vi "Publish.vi"(7 "Event Name":string, 8 "error in (no error)":errorcluster, 9 "Main Message":string="This text isn't used for sms", 10 "Subject":string="This is a test of the blah blah blah message system", 11 "connection in":T1) -> (0 "error out":errorcluster, 3 "connection out":T1)   [LabVIEW 2014, in "FRCts20_SNS.lvlib"]
uses:
  FRCts20_SNS.lvlib
  <vilib>/National Instruments/NI Amazon Web Services (AWS) Toolkit for LabVIEW/SNS/VI Source/AWS SNS Class/AWS_SNS.lvclass
  <vilib>/National Instruments/NI Amazon Web Services (AWS) Toolkit for LabVIEW/S3/vi source/Typedefs/AMZ_S3_AWS Credentials.ctl
  <vilib>/National Instruments/NI Amazon Web Services (AWS) Toolkit for LabVIEW/S3/vi source/LV Interface for Amazon S3.lvlib
  <vilib>/addons/database/NI_Database_API.lvlib
  <vilib>/addons/database/Connection.llb/DB Tools Open Connec (String).vi
  <vilib>/addons/database/Connection.llb/Conn ObjectReference.ctl
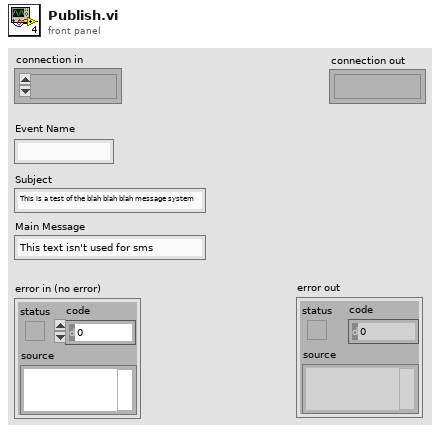
[diagram p1: front panel]
types:
  T1 = typedef "NI_Database_API.lvlib/Conn ObjectReference.ctl" = refnum<k1>
  T2 = typedef "LV Interface for Amazon S3.lvlib/AMZ_S3_AWS Credentials.ctl" = cluster{"Access Key":string, "Secret Key":string}
  T3 = cluster{string, "Subject":string, "TopicArn":string, "MessageStructure":string}
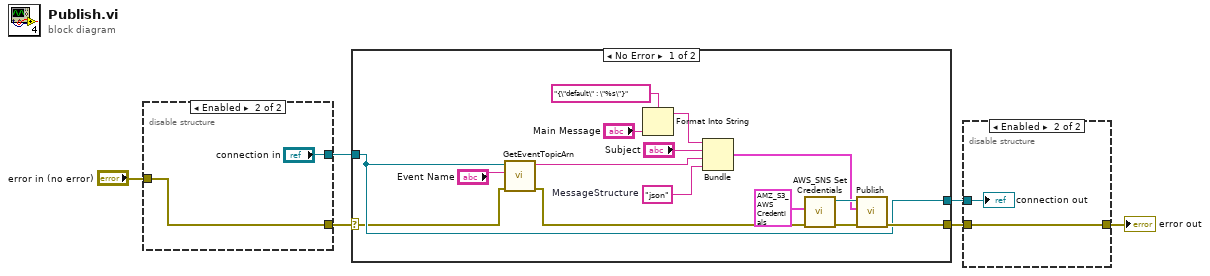
[diagram p0: block diagram]
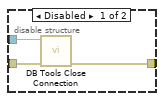
[diagram p2: hidden frame]
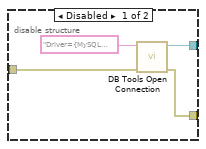
[diagram p3: hidden frame]
diagram:
  n1 = disable-structure shown="Enabled" {
    disable-tunnel: [w9 "connection in"] -> w6
    disable-tunnel: "error in (no error)" -> [w8 w12]
    disable-tunnel: [w7 w12] -> w4
    frame Disabled {
      n2 = call-poly <vilib>:"DB Tools Open Connection.vi"("error in (no error)"=w8, "connection information"="Driver={MySQL ODBC 5.2w Driver};Server=parkway-test-db.cjlclmebggwl.us-east-1.rds.amazonaws.com;Database=parkway;User=parkway;Password=moonlightmarj" ("Connection String")) -> ("error out"=w7:errorcluster, "connection reference"=w9:T1)  [unwired: 6 in]
    }
    frame Enabled {
    }
  }
  n3 = case shown="No Error" w4 {
    selector: w4 -> [w14 w29]
    tunnel: [w21 w29] -> w3
    tunnel: w6 -> [w15 w28]
    tunnel: [w15 w28] -> w1
    frame No Error {
      w24 = "json"  # MessageStructure
      n4 = call "GetEventTopicArn.vi"("error in (no error)"=w14, "Event Name"="Event Name", "Refnum in"=w15) -> ("error out"=w13:errorcluster, "TopicArn"=w16:string)  [unwired: 7 in]
      n5 = Format Into String(format string="{\"default\" : \"%s\"}" ("MessageFormat"), "Main Message") -> (resulting string=w18:string)  [unwired: 2 in, 1 out]
      n6 = Bundle(w18, "Subject"="Subject", "TopicArn"=w16, "MessageStructure"=w24) -> (w22:T3)  [unwired: 1 in]
      n7 = call <vilib>:"AWS_SNS Set Credentials.vi"("error in (no error)"=w13, "AWS Credentials"=T2 {"Access Key"="AKIAI4UOFGXQQ2XM3KTQ", "Secret Key"="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"} ("AWS Credentials in")) -> ("error out"=w23:errorcluster, "AWS_SNS.lvlib:AWS_SNS.lvclass"=w26:refnum<class "AWS_SNS.lvclass">)  [unwired: 8 in]
      n8 = call-dynamic "Publish.vi"("AWS_SNS in"=w26, "Publish Parameters"=w22, "error in (no error)"=w23) -> ("error out"=w21:errorcluster)  [unwired: 5 in, 2 out]
    }
    frame Error {
    }
  }
  n9 = disable-structure shown="Enabled" {
    disable-tunnel: w3 -> [w32 w34]
    disable-tunnel: [w31 w34] -> w2
    disable-tunnel: w1 -> [w30 w33]
    frame Disabled {
      n10 = call <vilib>:"DB Tools Close Connection.vi"("error in (no error)"=w32, "connection reference"=w30) -> ("error out"=w31:errorcluster)  [unwired: 5 in]
    }
    frame Enabled {
      "connection out" <- w33
    }
  }
  "error out" <- w2
